vi "RadCuerpoNegro.vi"() -> ()   [LabVIEW 2024]
uses:
  <vilib>/Waveform/WDTOps.llb/WDT Append Waveforms DBL.vi
  <vilib>/Waveform/WDTFileIO.llb/Export Waveform To Spreadsheet File.vi
  <instrlib>/Arduino UNO/Arduino UNO.lvlib
panel:
  out "Sensor 3":waveform(dbl)(graph)
  out "Sensor 1":waveform(dbl)(graph)
  out "Sensor 2":waveform(dbl)(graph)
  in  "stop":bool
  in  "VISA resource name":refnum<visa-resource-name>
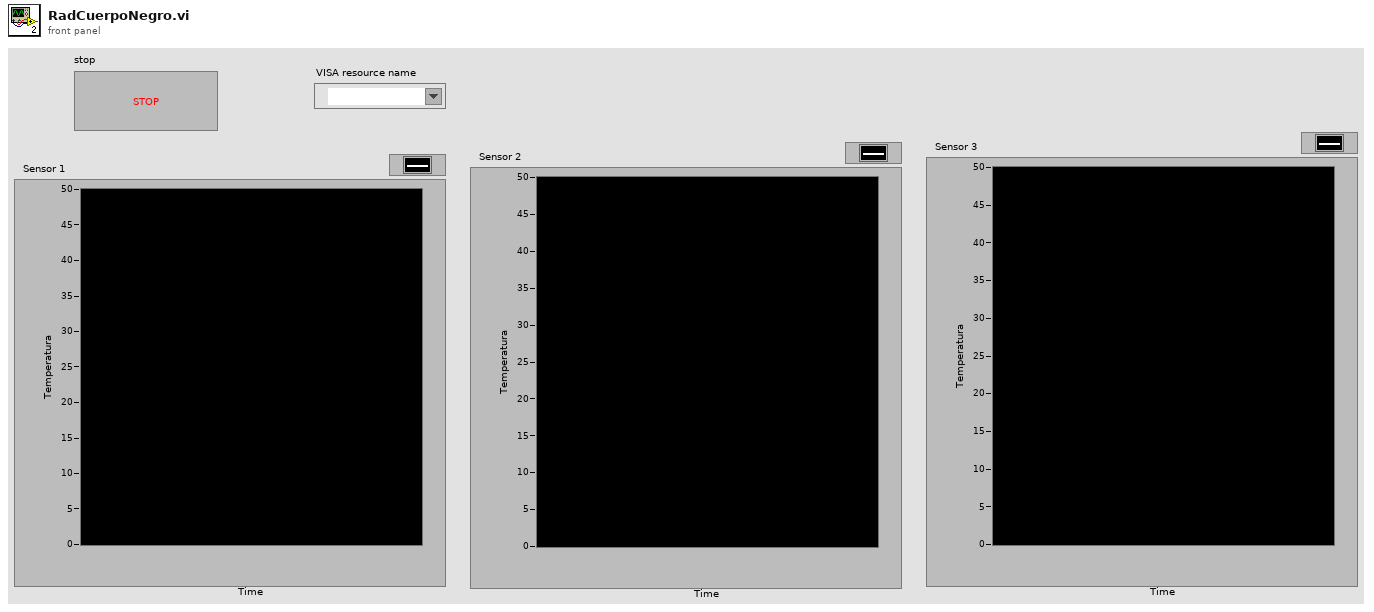
[diagram p1: front panel]
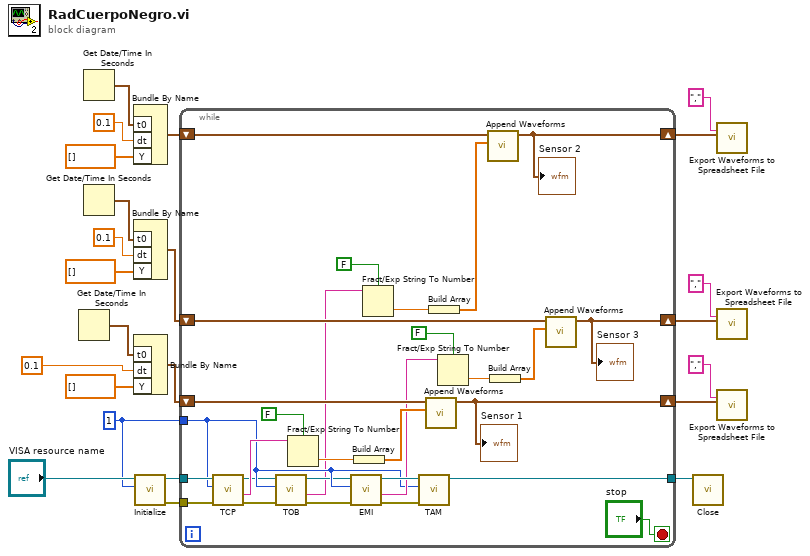
[diagram p0: block diagram]
diagram:
  w20 = u8 1 ("Address")
  n1 = Get Date/Time In Seconds() -> (seconds since 1Jan1904=w1:timestamp)
  n2 = Get Date/Time In Seconds() -> (seconds since 1Jan1904=w16:timestamp)
  n3 = Get Date/Time In Seconds() -> (seconds since 1Jan1904=w10:timestamp)
  n4 = Bundle By Name("t0"=w16, "dt"=0.1, "Y"=dbl[] []) -> (w15:waveform(dbl))  [unwired: 1 in]
  n5 = Bundle By Name("t0"=w10, "dt"=0.1, "Y"=dbl[] []) -> (w9:waveform(dbl))  [unwired: 1 in]
  n6 = Bundle By Name("t0"=w1, "dt"=0.1, "Y"=dbl[] []) -> (w8:waveform(dbl))  [unwired: 1 in]
  n7 = call <instrlib>:"Initialize.vi"("Address"=w20, "VISA resource name"="VISA resource name") -> ("error IO"=w22:errorcluster, "VISA resource name out"=w21:refnum<visa-resource-name>)  [unwired: 7 in, 1 out]
  n8 = while {
    tunnel: w22 -> [w34]
    tunnel: w21 -> [w35]
    tunnel: w20 -> [w28]
    tunnel: [w32] -> w19
    shift-right: [w43] -> w7
    shift-left: w15 -> [w45]
    shift-right: [w38] -> w5
    shift-left: w8 -> [w42]
    shift-right: [w37] -> w6
    shift-left: w9 -> [w41]
    stop <- "stop" stop-if-true
    n9 = call <instrlib>:"TCP.vi"("error in (no error)"=w34, "Address"=w28, "VISA resource name"=w35) -> ("error IO"=w33:errorcluster, "Tem LM"=w36:string, "VISA resource name out"=w27:refnum<visa-resource-name>)  [unwired: 6 in]
    n10 = call <instrlib>:"TOB.vi"("error in (no error)"=w33, "Address"=w28, "VISA resource name"=w27) -> ("error IO"=w25:errorcluster, "Temp Objeto"=w24:string, "VISA resource name out"=w26:refnum<visa-resource-name>)  [unwired: 6 in]
    n11 = Fract/Exp String To Number(use system decimal point (T)=FALSE, string=w36) -> (number=w47:dbl)  [unwired: 2 in, 1 out]
    n12 = call <instrlib>:"EMI.vi"("error in (no error)"=w25, "Address"=w28, "VISA resource name"=w26) -> ("error IO"=w29:errorcluster, "Emisividad"=w30:string, "VISA resource name out"=w31:refnum<visa-resource-name>)  [unwired: 6 in]
    n13 = Build Array(w47) -> (w39:dbl[])
    n14 = Fract/Exp String To Number(use system decimal point (T)=FALSE, string=w24) -> (number=w48:dbl)  [unwired: 2 in, 1 out]
    n15 = call <instrlib>:"TAM.vi"("error in (no error)"=w29, "Address"=w28, "VISA resource name"=w31) -> ("VISA resource name out"=w32:refnum<visa-resource-name>)  [unwired: 6 in, 2 out]
    n16 = call-poly <vilib>:"Append Waveforms.vi"("waveform B"=w39, "waveform A"=w42) -> ("waveform out"=w38:waveform(dbl))  [unwired: 8 in, 1 out]
    "Sensor 1" <- w38
    n17 = Build Array(w48) -> (w44:dbl[])
    n18 = Fract/Exp String To Number(use system decimal point (T)=FALSE, string=w30) -> (number=w49:dbl)  [unwired: 2 in, 1 out]
    n19 = call-poly <vilib>:"Append Waveforms.vi"("waveform B"=w44, "waveform A"=w45) -> ("waveform out"=w43:waveform(dbl))  [unwired: 8 in, 1 out]
    "Sensor 2" <- w43
    n20 = Build Array(w49) -> (w40:dbl[])
    n21 = call-poly <vilib>:"Append Waveforms.vi"("waveform B"=w40, "waveform A"=w41) -> ("waveform out"=w37:waveform(dbl))  [unwired: 8 in, 1 out]
    "Sensor 3" <- w37
  }
  n22 = call <instrlib>:"Close.vi"("VISA resource name"=w19) -> ()  [unwired: 10 in, 1 out]
  n23 = call-poly <vilib>:"Export Waveforms to Spreadsheet File.vi"("delimiter (Tab)"=",", "waveform"=w7) -> ()  [unwired: 8 in, 2 out]
  n24 = call-poly <vilib>:"Export Waveforms to Spreadsheet File.vi"("delimiter (Tab)"=",", "waveform"=w6) -> ()  [unwired: 8 in, 2 out]
  n25 = call-poly <vilib>:"Export Waveforms to Spreadsheet File.vi"("delimiter (Tab)"=",", "waveform"=w5) -> ()  [unwired: 8 in, 2 out]
